vi "blowfish_init.vi"(4 "error in (no error)":errorcluster, 7 "Key":string) -> (0 "error out":errorcluster, 2 "S 4X256":u32[][](array[numeric]), 3 "P 18":u32[](array[numeric]))   [LabVIEW 2020]
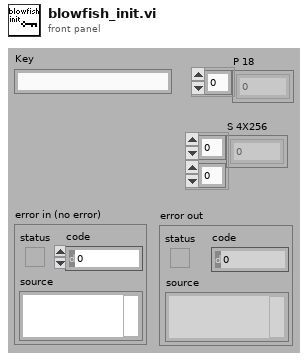
[diagram p1: front panel]
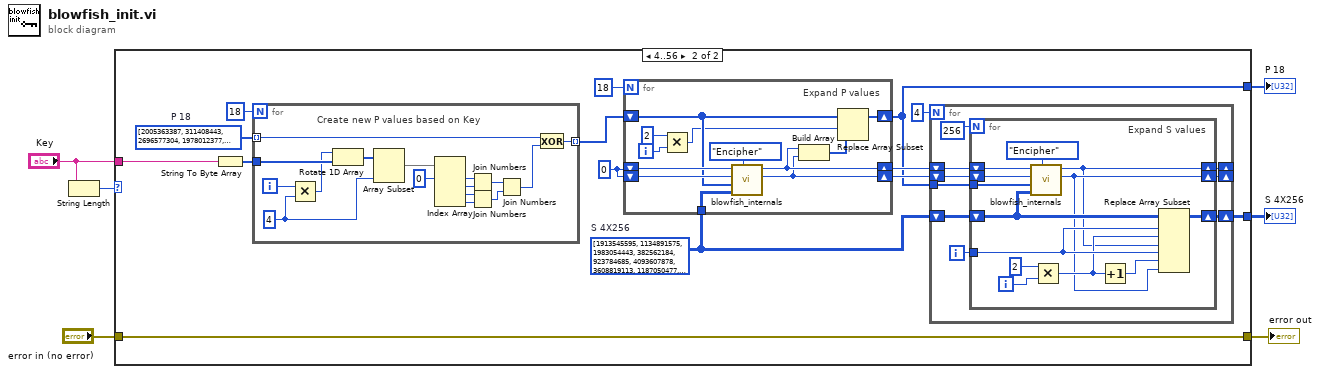
[diagram p0: block diagram]
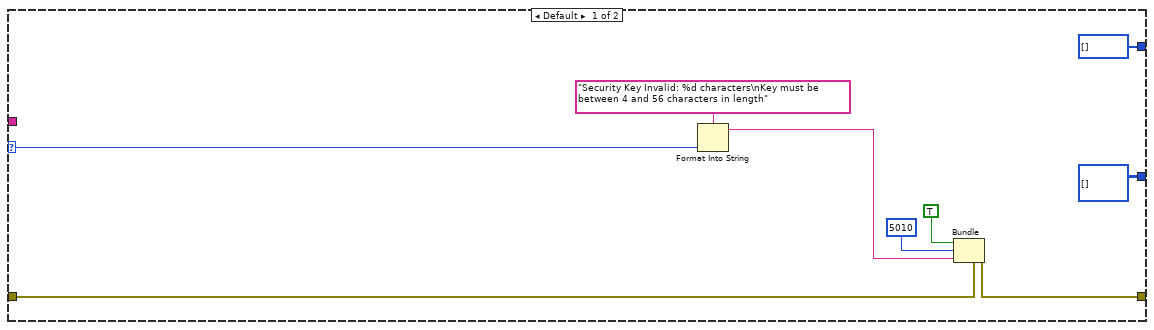
[diagram p2: hidden frame]
diagram:
  n1 = String Length(string="Key") -> (length=w4:i32)
  n2 = case shown="4..56" w4 {
    selector: w4 -> [w12 _]
    tunnel: "Key" -> [_ w28]
    tunnel: [u32[][] [] ("S 4X256") w19] -> w6
    tunnel: [u32[] [] w17] -> w5
    tunnel: "error in (no error)" -> [w11 w16]
    tunnel: [w10 w16] -> w1
    frame Default {
      n3 = Format Into String(format string="Security Key Invalid: %d characters\nKey must be between 4 and 56 characters in length" ("Halt Message"), w12) -> (resulting string=w8:string)  [unwired: 2 in, 1 out]
      n4 = Bundle(cluster=w11, "status"=TRUE ("Halt?"), "code"=5010 ("Halt Code"), "source"=w8) -> (w10:errorcluster)
    }
    frame 4..56 {
      w24 = u32 0
      w18 = u32[][] [[1913545595, 1134891575, 1983054443, 382562184, 923784685, 4093607878, 3608819113, 1187050477, 1441899992, 4067036799, 2501846090, 3549933725, 811886515, 2049793556, 376862373, 1741112599, 2856873639, 2463427364, 623872356, 2015562173, 350679356, 1297549870, 4263767100, 106844521, 3040223950, 716548635, 4135339846, 2204216277, 3564108977, 1440906251, 3389789163, 1735815772, 1076034989, 3751743627, 2813280960, 2623479024, 3463752843, 3903330551, 821992440, 4063483229, 3097980760, 4205336644, 1141710392, 2277477913, 2615784896, 1094867784, 1000659620, 967508157, 2953319782, 939984335, 2879101359, 753111570, 592973794, 3346319043, 3630687139, 391718102, 315371064, 1705599382, 355141432, 11531844, 2064975857, 3504427308, 2858892507, 2577170886, 1951152364, 1802478074, 516768395, 2091633832, 3010796997, 914858570, 2478047302, 3204056173, 1652070002, 2652307402, 1560212147, 3384382167, 1478955766, 3584399434, 2990163407, 708961027, 3131321654, 1486911018, 640234461, 4121156384, 1936169560, 2588881432, 1410842727, 1599751816, 4041274537, 4148098597, 2000557116, 261096087, 3293328601, 2457351778, 3072753982, 664625121, 1145233021, 2934759568, 1022407097, 3680952106, 3439174052, 4174301791, 275022380, 3972169916, 357748573, 3847534447, 3326082841, 2274087143, 317287736, 2320473793, 3119596895, 1447794793, 3756256429, 277136987, 2120856181, 1848831619, 580603909, 3322458831, 3870808958, 4036847755, 3637505964, 2088079419, 609839900, 4142362225, 3338187822, 2969047790, 4248325633, 2943807287, 222086796, 2100868995, 4247267184, 3485600712, 2494084171, 213243610, 2109641929, 3043149422, 221882761, 196510686, 2605948138, 757033274, 3545213499, 799763668, 3903298729, 2039339989, 412098806, 1059736753, 226652798, 1004343567, 2181201797, 405923303, 4058918593, 1359586062, 2317491325, 1266082950, 239892874, 3857224749, 4058279676, 2816876004, 2555978827, 1162899330, 3520491292, 3460021455, 2402388479, 3334633241, 4125781199, 1076227943, 599651896, 3714190197, 275430186, 872078836, 3602139662, 1044781839, 1690056017, 1204639822, 1650547302, 1733361443, 1950077019, 320340192, 824806428, 2300485571, 3803804018, 3292224465, 2517031040, 2422470384, 3578310944, 1959803478, 3290838173, 857037534, 3224862886, 615239298, 1220388553, 3352264313, 4246127459, 3694093473, 3878065951, 257525514, 3629650050, 4220748954, 369705285, 57860017, 672662026, 1235085019, 2236559950, 3431123249, 3467534366, 1082557305, 3694448658, 1092942993, 403471379, 2051951326, 1681427507, 72190751, 915279460, 833365152, 639740654, 556226390, 2085647474, 34690421, 3707859061, 2418179226, 3446702509, 2440173355, 217735257, 1888781447, 2773799416, 926477604, 3696269520, 2152895407, 3268268760, 979146758, 1924059650, 367583945, 29320571, 4066345354, 3442448313, 2505755771, 2653045693, 4255962025, 128914036, 2981426301, 2492241505, 1861323815, 1365793046, 3535124880, 1010138147, 1425361023, 1092503211, 3687128122, 2466700235, 3755403061, 960251841, 3818090347, 613107146, 1174838745, 2891029609, 1638781544], [3818939239, 1699513110, 3127354028, 1324946801, 4187222736, 3768883807, 2525264099, 1856402133, 2056430722, 1665916266, 700397213, 9527428, 2010652963, 3495560594, 502603918, 230799970, 395322394, 2256069354, 210563560, 2138334540, 3369181486, 3483646806, 812249411, 1558810618, 3824324989, 1290816485, 2269652799, 3019207103, 4246861910, 3028757039, 2035280484, 2324801890, 508967899, 2551182510, 4267116066, 1333929544, 1871015888, 4084861914, 450784470, 436004754, 535508388, 1566084682, 841078607, 3596852537, 3151624146, 1649164026, 3012744396, 1778423053, 467836775, 1966816667, 1324563927, 1088815128, 4186313318, 1001451814, 1299484321, 142184925, 2244008159, 3662400923, 3380037070, 1788988896, 4230378907, 1243771163, 2830628941, 3490173228, 3745436051, 3978643435, 3006742944, 4032935155, 1144352053, 3771623563, 2783889020, 1065257868, 619939519, 2588730437, 3722218612, 1907150675, 687756046, 53444814, 43451127, 3239004846, 4211240386, 3416591577, 3991047958, 1083378162, 1408944664, 1137640590, 3343567130, 1928503628, 1366491148, 1483164155, 3642610373, 1214171177, 138422203, 3254954685, 2549476653, 3365323415, 2466807711, 154780470, 3218129567, 1288453031, 2249783433, 3173130474, 2661013910, 1341121295, 3554069061, 3959748305, 4028417735, 2543463112, 3815221906, 1943298671, 2937375925, 1181178344, 577028358, 1421621961, 1064128317, 3967435813, 331247575, 964909876, 1297937149, 2269369541, 2397471023, 3113000872, 2374247897, 2026653686, 96386429, 2930736267, 3484667182, 3000001660, 3081580466, 1109480602, 2850844930, 3106939599, 2474021690, 1162184602, 2222622569, 3520210255, 2150067538, 2559356225, 242802151, 1646906497, 2536134443, 2523811583, 381236914, 1190090125, 1777668999, 1545702261, 3768478284, 1548942184, 3956757890, 1156505773, 2147163579, 3073360501, 2536797010, 1875789911, 1129423500, 1967511027, 1698171068, 3564719870, 4180664312, 1302845945, 1300094043, 3882466831, 2150596430, 3306247053, 2560491305, 2406952034, 1990041142, 1492301840, 1779687645, 2495859499, 3903697632, 1855432271, 920550455, 1048170857, 312880278, 59299652, 2295729454, 4062654941, 2163674640, 2177383635, 280843799, 2951592679, 2280872109, 1357657712, 2534539093, 989397837, 3923064002, 1649912480, 3867842012, 3417589351, 4052051555, 2391755991, 734007898, 3659011453, 3701631598, 1609728851, 2292161718, 3891971390, 2236289422, 1475905710, 3473756265, 1246839464, 2095590091, 2514688587, 1279653958, 929459362, 3708802157, 2057313436, 3653243109, 3995540334, 4215535095, 3697355031, 2339977626, 2117734004, 2049758674, 1044753334, 2326449231, 2828070539, 79725457, 3194732847, 1136641838, 3691500282, 3165067470, 2504389124, 405279990, 3049745165, 4067287430, 3530125663, 1536015805, 2216539469, 2453700051, 264332751, 955605512, 1812115909, 2120486772, 728165013, 1251883941, 355696979, 2316884255, 226135218, 2073310430, 3122626197, 1314040083, 1696477871, 2137292033, 90725530, 688915644, 487712510, 2813713208, 3557155455, 2343039544, 1855100246, 188883402, 1460603629, 1129327462, 3971410966], [1622580199, 1602539068, 2880514582, 1931877528, 1168845047, 3002392493, 3353098979, 1961568464, 996487814, 3177713235, 3638418932, 2211555943, 3066516174, 1928002653, 53449272, 3294850527, 2446997200, 1824957367, 683061346, 329332296, 397532585, 3391733642, 943618040, 1980870873, 1407289930, 2611132093, 1856591130, 2543014655, 3714984021, 3171257184, 4077089801, 698822190, 1449738414, 555904411, 3439106347, 3196976885, 4015912711, 3510575155, 2772837683, 4127030028, 903914178, 973546861, 1359577851, 3880779452, 2612214500, 510574980, 814009152, 1151773857, 3058723030, 2487116882, 3988940293, 3470332982, 3840833260, 2817314865, 1401496984, 2867718451, 3008511353, 4267888248, 3911015031, 1374860481, 3988302473, 2585259739, 4048632653, 2396245140, 2922861616, 2665860897, 3673344249, 2477867491, 3532757401, 3205793173, 2489960419, 2991550882, 3612083440, 410408411, 1619904920, 3518449900, 94224073, 3078601593, 4277424594, 3305757238, 1316659953, 223733323, 3351189161, 738200797, 2320503325, 4000197286, 454314670, 782833985, 4207379091, 1105251007, 683391980, 2381521780, 3525941827, 1907814813, 509003604, 3806754352, 2655619875, 1283608100, 360127041, 3080366991, 4223312772, 1883542570, 811427258, 1958821008, 82974241, 3545596445, 838984492, 915310656, 2064395674, 2864595977, 66644456, 2794778400, 2104095595, 2142927432, 2088421488, 1684847056, 1720423340, 3021217802, 2050737669, 2600892690, 3419359157, 3860850874, 3936158020, 3038024036, 985414923, 1032858449, 3798446975, 1900873332, 3642302490, 2146789032, 2630028415, 3297069358, 3726406887, 2228499824, 3498792579, 1828819863, 712569570, 208815412, 3940686522, 3407756282, 732326248, 3675951973, 1095101579, 2342701319, 2143880701, 2569312332, 3765177865, 3912190680, 257734022, 3207892042, 1717107840, 797071528, 642777511, 3132529427, 14717350, 2281223057, 1695322110, 199269040, 2071353594, 965443948, 2380491932, 3474455883, 3071927278, 1929275117, 1204077221, 1489492091, 2982761762, 2243348409, 2794372311, 3290961498, 505739610, 1146657477, 3641204433, 3823882266, 274486498, 152637564, 2223686131, 3906881781, 3865181484, 3602286275, 959029193, 2340993953, 1161992292, 3984108464, 2186044485, 3640665499, 3398845285, 3548740555, 473875499, 2638859971, 1780775155, 4025794298, 1993966897, 2656877440, 2140519014, 213916506, 1746346600, 1796342227, 3157737318, 141965123, 960183811, 2584800437, 348053851, 2424895184, 53868012, 590118502, 743619474, 3347967626, 1570110194, 2536746688, 1194204032, 2916250667, 989150105, 3839576314, 3667547259, 2990115196, 1473595900, 836079866, 2873461807, 2610472712, 2086980354, 1927334725, 2648567139, 3700067349, 345983066, 1416376332, 2457237211, 866124990, 3508094481, 1072163372, 11599459, 1164515445, 6293656, 3829613815, 1584749178, 1147918675, 1093677336, 3453394443, 3039618774, 1919851830, 3980038897, 4086725324, 2193172771, 1192636322, 3006415551, 3891474882, 1837009236, 370022728, 1762422483, 2978543589, 313343714, 3815792845, 129895862, 2812028613, 4144939476, 1026019591], [3106846321, 2426021924, 3852192696, 410580026, 2218273391, 3660001192, 2677093828, 1090934087, 1103468935, 1786717135, 2188417639, 2580972158, 1599223044, 2852067465, 423381285, 1395888359, 554200656, 336037308, 4062709930, 1427937247, 1920888568, 3421193847, 476414677, 1655546636, 2338159558, 1734595360, 3012433593, 2236562252, 3713950832, 2069657848, 3812054192, 1623563747, 1530712575, 3361231154, 1887351055, 3720295388, 3372596897, 2819758123, 1794173515, 1755651568, 1327131086, 4125048654, 4203150662, 1098491480, 281478490, 4261193459, 1538352008, 1890539867, 1825386492, 3189159439, 3432589722, 4041538116, 3688763337, 3958461122, 2753646622, 867707775, 97209577, 2846937093, 349990096, 4157250741, 2119664502, 4038707872, 1017399343, 1914794916, 1687862114, 1856644989, 3451567199, 1767501515, 1206404886, 324688647, 150243679, 459865116, 3484827529, 631471855, 1783770253, 701718967, 3880981719, 1449172090, 534920057, 3311669911, 1707005575, 3324708385, 3540644762, 2582249795, 2606042602, 221676090, 450041385, 2399828341, 1234423096, 2546565202, 1475855533, 1530771595, 1730356750, 1307239801, 3715323896, 2119800135, 2036710955, 2794528786, 2467932124, 1027339049, 3546604348, 2316968530, 1071126450, 278166578, 845356284, 1266821049, 3502454496, 3625171496, 110801016, 71426724, 3616415762, 2509357192, 2799941938, 3496234296, 1643556861, 3448132916, 895964632, 373784922, 468007857, 1601473368, 3475583213, 1824179942, 1502564650, 2684457896, 1997718755, 3475514214, 1213061676, 347438352, 1616457466, 3939542297, 2374563453, 3932032984, 431219902, 1011621758, 1830695739, 4283910591, 4178615003, 1628927336, 3745815025, 333407614, 1790977922, 2407191245, 3655408793, 4275501954, 429841488, 986290619, 740476391, 1218600094, 828781876, 4213188513, 2666622316, 3778721313, 2872899997, 3555788746, 4169499105, 681722076, 2487672377, 2069082775, 712721431, 217893511, 72781676, 1698162546, 4266667210, 3401593237, 3468288393, 1071218499, 1604760367, 1821825056, 2728323825, 2994090086, 720776049, 2192842912, 2068639580, 602532527, 1246953637, 63958077, 1049518334, 2056772178, 1394298427, 1254843559, 2133418313, 1382948325, 3145938388, 2896394699, 4176985936, 2017398276, 3874720723, 1741122608, 146517015, 3485200728, 3669381654, 397687292, 2446366832, 1938932936, 3231352074, 4092079150, 3584706145, 149763510, 478682716, 1010594168, 1313712900, 2934132799, 4213028746, 2506466534, 1452535303, 2557318155, 90244120, 1159628762, 523311275, 1259628010, 1213145887, 2368695887, 154696389, 2415804142, 1899026833, 2065727111, 1903046330, 2806277388, 93675386, 1188339444, 1781216831, 1593370962, 871169596, 1570138371, 844495548, 1757762265, 2710223353, 1221356550, 2216984887, 297858716, 2634790612, 1716865594, 2656578243, 1752975640, 2486135163, 1843488370, 1755568293, 156988020, 2525228596, 38092714, 1352325, 872433495, 3130965361, 4044629207, 2797667142, 1777238288, 2808185155, 1441396684, 4293506486, 1535876935, 1951339276, 1102222092, 2161573525, 2647673150, 1365538834, 2888307026]]  # S 4X256
      w26 = u32[] [2005363387, 311408443, 2696577304, 1978012377, 4042222433, 722114356, 802677996, 4256358732, 1985170914, 473917298, 1415250683, 4081676184, 2783414768, 3627112570, 1753927079, 903846569, 1967614054, 1094009069]  # P 18
      n5 = String To Byte Array(string=w28) -> (unsigned byte array=w27:u8[])
      n6 = for {
        N: 18 -> [_]
        tunnel: w27 -> [w68]
        tunnel: w26 -> [w70] mode=indexing
        tunnel: [w69] -> w25 mode=indexing
        i -> [w64]
        w65 = 4 ("length")
        # "Create new P values based on Key"
        n7 = Multiply(x=w64, y=w65) -> (x*y=w66:i32)
        n8 = Rotate 1D Array(1:w68, 2:w66) -> (0:w67:u8[])
        n9 = Array Subset(array=w67, length=w65) -> (w79:u8[])  [unwired: 1 in]
        n10 = Index Array(array=w79, index #1=0 ("index")) -> (element #1=w77:u8, element #2=w76:u8, element #3=w75:u8, element #4=w74:u8)  [unwired: 3 in]
        n11 = Join Numbers(hi=w77, lo=w76) -> ((hi.lo)=w73:u16)
        n12 = Join Numbers(hi=w75, lo=w74) -> ((hi.lo)=w72:u16)
        n13 = Join Numbers(hi=w73, lo=w72) -> ((hi.lo)=w71:u32)
        n14 = Exclusive Or(1:w71, 2:w70) -> (0:w69:u32)
      }
      n15 = for {
        N: 18 -> [_]
        shift-right: [w54] -> w17
        shift-left: w25 -> [w61]
        shift-right: [w60] -> w21
        shift-left: w24 -> [w63]
        shift-right: [w59] -> w20
        shift-left: w24 -> [w62]
        tunnel: w18 -> [w53]
        i -> [w58]
        # "Expand P values"
        n16 = Multiply(x=2, y=w58) -> (x*y=w56:i32)
        n17 = call "blowfish_internals.vi"("Enc/Dec"=enum16{"Encipher", "Decipher"}."Encipher", "S 4X256"=w53, "P 18"=w61, "Xr"=w62, "Xl"=w63) -> ("Xr out"=w59:u32, "Xl out"=w60:u32)  [unwired: 2 in]
        n18 = Build Array(w60, w59) -> (w52:u32[])
        n19 = Replace Array Subset(array=w61, new element=w52, index=w56) -> (w54:u32[])
      }
      n20 = for {
        N: 4 -> [_]
        shift-right: [w36] -> w19
        shift-left: w18 -> [w37]
        shift-right: [w33] -> _
        shift-left: w21 -> [w35]
        shift-right: [w32] -> _
        shift-left: w20 -> [w34]
        tunnel: w17 -> [w31]
        i -> [w30]
        n21 = for {
          N: 256 -> [_]
          shift-right: [w41] -> w36
          shift-left: w37 -> [w47]
          shift-right: [w39] -> w33
          shift-left: w35 -> [w49]
          shift-right: [w40] -> w32
          shift-left: w34 -> [w50]
          tunnel: w31 -> [w51]
          tunnel: w30 -> [w44]
          i -> [w45]
          # "Expand S values"
          n22 = call "blowfish_internals.vi"("Enc/Dec"=enum16{"Encipher", "Decipher"}."Encipher", "S 4X256"=w47, "P 18"=w51, "Xr"=w50, "Xl"=w49) -> ("Xr out"=w40:u32, "Xl out"=w39:u32)  [unwired: 2 in]
          n23 = Multiply(x=2, y=w45) -> (x*y=w42:i32)
          n24 = Increment(x=w42) -> (x+1=w43:i32)
          n25 = Replace Array Subset(array=w47, new element #1=w39, index (row) #1=w44, index (col) #1=w42, new element #2=w40, index (row) #2=w44, index (col) #2=w43) -> (w41:u32[][])
        }
      }
    }
  }
  "S 4X256" <- w6
  "P 18" <- w5
  "error out" <- w1
